vi "Read.vi"(6 "Append Index":i32, 8 "error in (no error)":errorcluster, 11 "Data.TDMS":refnum<class "Data.TDMS.lvclass">) -> (0 "error out":errorcluster, 1 "Notes":string, 2 "Data (Dictionary)":T1[](array[typedef]), 3 "Data.TDMS out":refnum<class "Data.TDMS.lvclass">, 5 "Path out":path)   [LabVIEW 2016, in "Data.TDMS.lvclass"]
uses:
  Data.TDMS.lvclass
  C:/user/patrick/git/LV-to-ITX/src/Data/Data.lvclass
  Data/Typedefs/Dictionary--cluster.ctl
  Data.TDMS.lvclass/Data.TDMS.ctl
  Data/Data.lvclass/Data.ctl
  Data/Data.lvclass
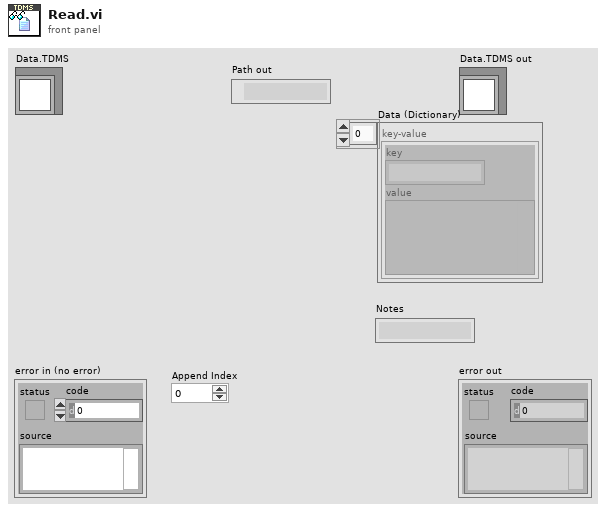
[diagram p1: front panel]
types:
  T1 = typedef "Data.lvclass/Dictionary--cluster.ctl" = cluster{"key":string, "value":variant}
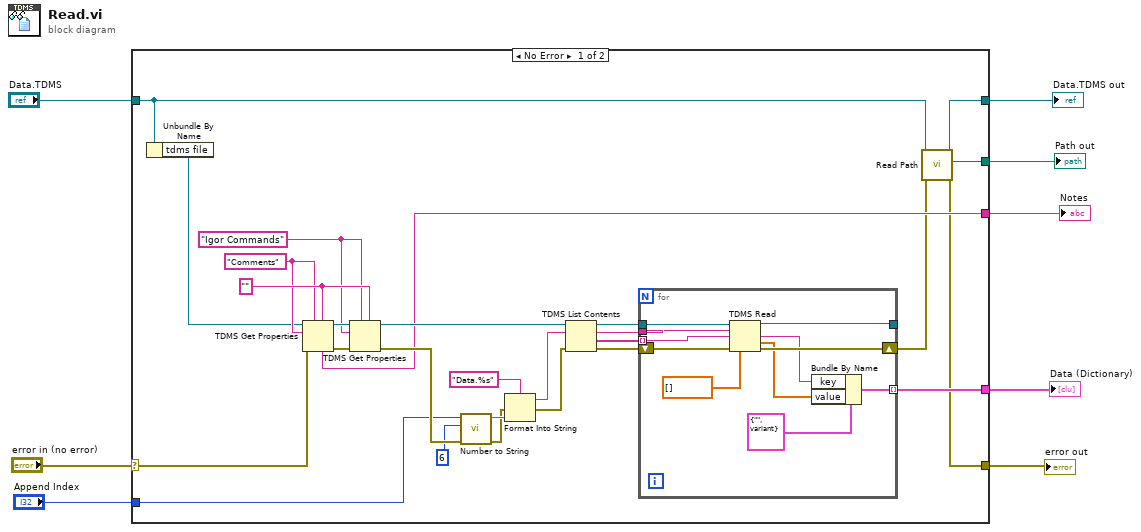
[diagram p0: block diagram]
diagram:
  n1 = case shown="No Error" "error in (no error)" {
    selector: "error in (no error)" -> [w9 w47]
    tunnel: "Data.TDMS" -> [w13 w46]
    tunnel: [w14 w46] -> w7
    tunnel: [w11 w47] -> w6
    tunnel: [w15 _] -> w5
    tunnel: "Append Index" -> [w18 _]
    tunnel: [w17 _] -> w3
    tunnel: [w16 _] -> w2
    frame No Error {
      w35 = "" ("attrib name")
      w28 = "Igor Commands" ("attrib name")
      w29 = "Comments" ("attrib name")
      n2 = Unbundle By Name(w13) -> ("tdms file"=w10:refnum<k34>)
      n3 = TDMS Get Properties(5:w35, 7:w29, 8:w9, 10:w29, 11:w10) -> (0:w32:errorcluster, 3:w33:refnum<k34>, 4:w17:string)  [unwired: 1 in, 3 out]
      n4 = TDMS Get Properties(5:w35, 7:w28, 8:w32, 10:w28, 11:w33) -> (0:w21:errorcluster, 3:w34:refnum<k34>)  [unwired: 1 in, 4 out]
      n5 = call <userlib>:"Number to String.vi"("error in (no error)"=w21, "desired minimum string length"=6, "number"=w18) -> ("error out"=w20:errorcluster, "String"=w25:string)  [unwired: 7 in]
      n6 = Format Into String(format string="Data.%s", error in=w20, w25) -> (resulting string=w24:string, error out=w22:errorcluster)  [unwired: 1 in]
      n7 = TDMS List Contents(4:w22, 6:w24, 7:w34) -> (0:w30:errorcluster, 1:w26:string[], 2:w27:string, 3:w31:refnum<k34>)
      n8 = for {
        shift-right: [w42] -> w12
        shift-left: w30 -> [w45]
        tunnel: w26 -> [w37] mode=indexing
        tunnel: w27 -> [w41]
        tunnel: [w40] -> w16 mode=indexing
        tunnel: w31 -> [w43]
        tunnel: [w44] -> _
        n9 = TDMS Read(0:w43, 5:w41, 7:w37, 11:w45, 12:dbl[] [] ("array type (2D Dbl)")) -> (4:w44:refnum<k34>, 10:w36:dbl[], 15:w42:errorcluster)  [unwired: 3 in, 3 out]
        n10 = Bundle By Name(cluster=T1 {"key"="", "value"=variant} ("key-value"), "key"=w37, "value"=w36) -> (w40:T1)
      }
      n11 = call "Read Path.vi"("error in (no error)"=w12, "Data Save"=w13) -> ("error out"=w11:errorcluster, "Path"=w15:path, "Data Save out"=w14:refnum<class "Data.TDMS.lvclass">)  [unwired: 7 in]
    }
    frame Error {
    }
  }
  "error out" <- w6
  "Data.TDMS out" <- w7
  "Path out" <- w5
  "Data (Dictionary)" <- w2
  "Notes" <- w3
